vi "Get Path Transformations.vi"(8 "error in (no error)":errorcluster, 11 "SDIST in":refnum<class "NI_AB_API_SDIST.lvclass">) -> (0 "error out":errorcluster, 1 "New Paths":path[](array[path]), 2 "Original Paths":path[](array[path]), 3 "SDIST out":refnum<class "NI_AB_API_SDIST.lvclass">)   [LabVIEW 2020, in "NI_AB_API_SDIST.lvclass"]
uses:
  <vilib>/AppBuilder/AB_API/SDIST/NI_AB_API_SDIST.lvclass
  <vilib>/AppBuilder/AB_API/Build/NI_AB_API_Build.lvclass
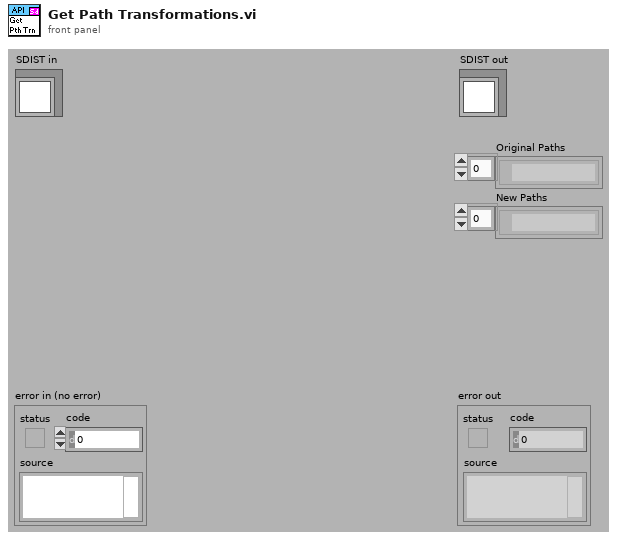
[diagram p1: front panel]
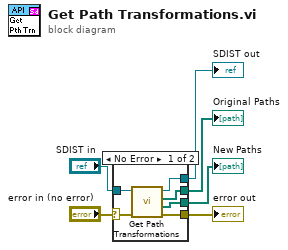
[diagram p0: block diagram]
diagram:
  n1 = case shown="No Error" "error in (no error)" {
    selector: "error in (no error)" -> [w10 w14]
    tunnel: [w9 w14] -> w5
    tunnel: [w11 w13] -> w3
    tunnel: "SDIST in" -> [w12 w13]
    tunnel: [w7 _] -> w2
    tunnel: [w8 _] -> w1
    frame No Error {
      n2 = call-parent "Get Path Transformations.vi"("error in (no error)"=w10, "NI_AB_API_Build in"=w12) -> ("error out"=w9:errorcluster, "New Paths"=w8:path[], "Original Paths"=w7:path[], "NI_AB_API_Build out"=w11:refnum<class "NI_AB_API_SDIST.lvclass">)  [unwired: 6 in]
    }
    frame Error {
    }
  }
  "error out" <- w5
  "SDIST out" <- w3
  "Original Paths" <- w2
  "New Paths" <- w1
